vi "Write WorkerMessages.vi"(8 "error in (no error)":errorcluster, 10 "Worker Messages":T1(array[cluster]), 11 "CS++PVProxy in":refnum<class "CS++PVProxy.lvclass">) -> (0 "error out":errorcluster, 3 "CS++PVProxy out":refnum<class "CS++PVProxy.lvclass">)   [LabVIEW 2015, in "CS++PVProxy.lvlib" / "CS++PVProxy.lvclass"]
uses:
  CS++PVProxy.lvclass
  CS++PVMonitor Messages/CS++PVUpdate Msg/CS++PVUpdate Msg.lvclass
  Classes/CS++ProcessVariables/PVConnection/PVConnection.lvclass
  CS++PVProxy.lvclass/CS++PVProxy.ctl
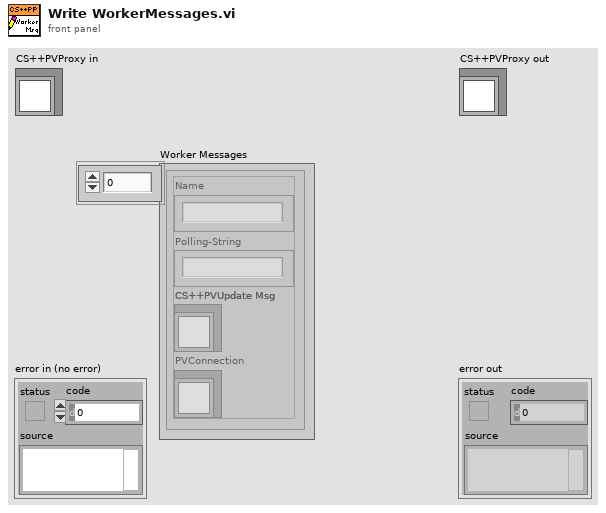
[diagram p1: front panel]
types:
  T1 = cluster{"Name":string, "Polling-String":string, "CS++PVUpdate Msg":refnum<class "CS++PVUpdate Msg.lvclass">, "PVConnection":refnum<class "PVConnection.lvclass">}[]
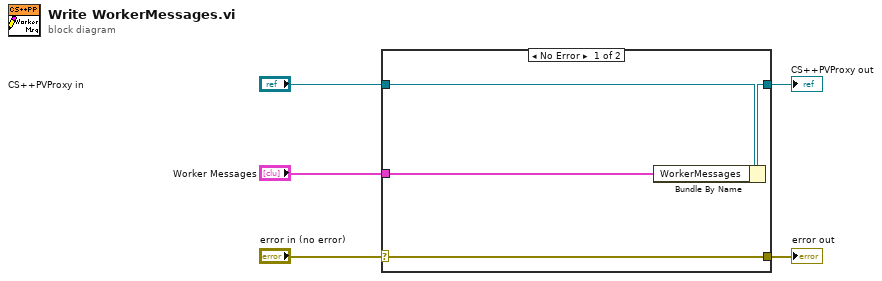
[diagram p0: block diagram]
diagram:
  n1 = case shown="No Error" "error in (no error)" {
    selector: "error in (no error)" -> [w9 w10]
    tunnel: [w9 w10] -> w4
    tunnel: [w7 w11] -> w2
    tunnel: "CS++PVProxy in" -> [w8 w11]
    tunnel: "Worker Messages" -> [w6 _]
    frame No Error {
      n2 = Bundle By Name(cluster=w8, "WorkerMessages"=w6) -> (w7:refnum<class "CS++PVProxy.lvclass">)
    }
    frame Error {
    }
  }
  "error out" <- w4
  "CS++PVProxy out" <- w2
